vi "Validate XYZ limits.vi"(0 "X":sgl format="%.3g", 5 "Y":sgl format="%.3g", 7 "Z":sgl format="%.3g", 9 "Action":enum16{"Set Limit", "Validate limit"}(ring)=enum."Validate limit", 11 "error in (no error)":errorcluster, 12 "Controller ID":T1) -> (4 "Limit ok":bool, 15 "error out":errorcluster)   [LabVIEW 2024, in "GRBL 1.1.lvlib"]
doc: "This VI validate if new position requested is outside the limits."
uses:
  GRBL 1.1.lvlib
  Controller ID.ctl
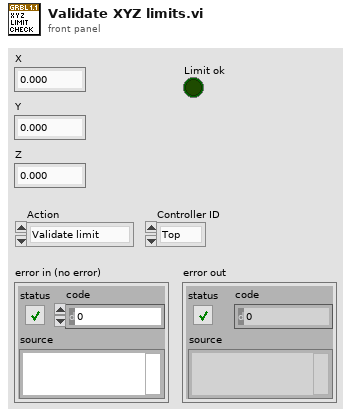
[diagram p1: front panel]
types:
  T1 = typedef "GRBL 1.1.lvlib/Controller ID.ctl" = enum16{"Top", "Bottom"}
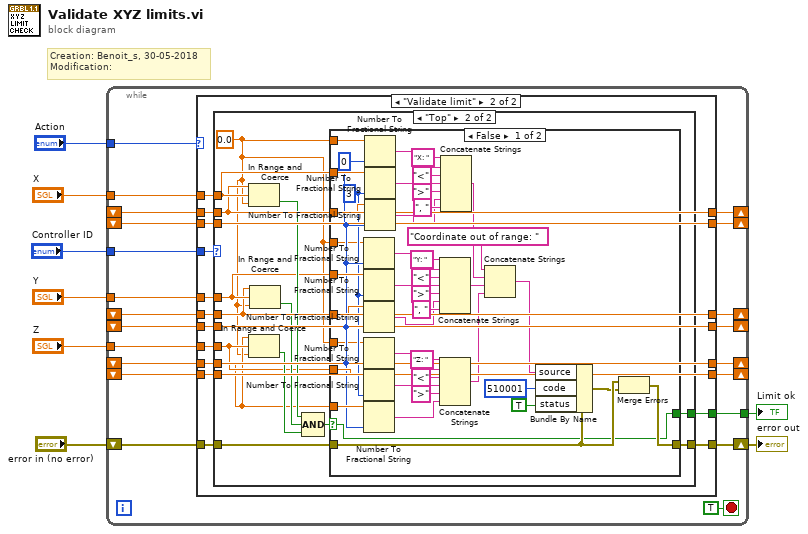
[diagram p0: block diagram]
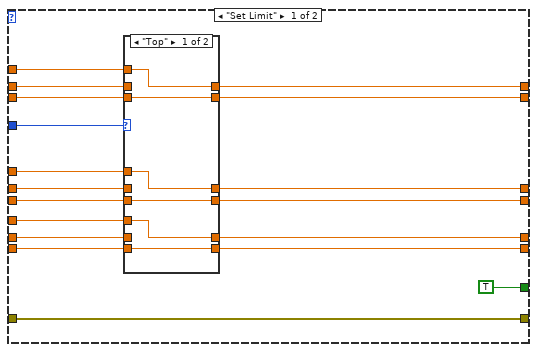
[diagram p2: hidden frame]
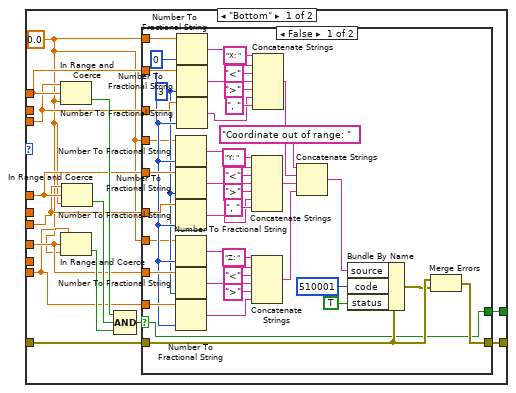
[diagram p4: hidden frame]
diagram:
  # "Creation: Benoit_s, 30-05-2018\nModification:"
  n1 = while {
    tunnel: "X" -> [w27]
    tunnel: "Y" -> [w26]
    tunnel: "Z" -> [w25]
    shift-right: [w28] -> w7
    shift-left: "error in (no error)" -> [w29]
    tunnel: [w23] -> w3
    tunnel: "Action" -> [w22]
    shift-right: [w18] -> _
    shift-left: _ -> [w21]
    shift-right: [w17] -> _
    shift-left: _ -> [w19]
    shift-right: [w16] -> _
    shift-left: _ -> [w20]
    tunnel: "Controller ID" -> [w15]
    shift-right: [w9] -> _
    shift-left: _ -> [w14]
    shift-right: [w10] -> _
    shift-left: _ -> [w13]
    shift-right: [w11] -> _
    shift-left: _ -> [w12]
    stop <- TRUE stop-if-true
    n2 = case shown="\"Validate limit\"" w22 {
      tunnel: w29 -> [w46 w72]
      tunnel: [w46 w71] -> w28
      tunnel: w27 -> [w43 w70]
      tunnel: w26 -> [w35 w69]
      tunnel: w25 -> [w33 w68]
      tunnel: [TRUE w67] -> w23
      tunnel: w21 -> [w32 w66]
      tunnel: w20 -> [w30 w64]
      tunnel: w19 -> [w31 w65]
      tunnel: [w44 w66] -> w18
      tunnel: [w36 w65] -> w17
      tunnel: [w34 w64] -> w16
      tunnel: w15 -> [w45 w63]
      tunnel: w14 -> [w37 w62]
      tunnel: w13 -> [w40 w61]
      tunnel: w12 -> [w41 w60]
      tunnel: [w42 w60] -> w11
      tunnel: [w39 w61] -> w10
      tunnel: [w38 w62] -> w9
      frame "Set Limit" {
        n3 = case shown="\"Top\"" w45 {
          tunnel: [w53 w58] -> w44
          tunnel: w43 -> [w53 w59]
          tunnel: [w52 w59] -> w42
          tunnel: w41 -> [w52 _]
          tunnel: w40 -> [w51 _]
          tunnel: [w51 w55] -> w39
          tunnel: [w50 w54] -> w38
          tunnel: w37 -> [w50 _]
          tunnel: [w49 w57] -> w36
          tunnel: w35 -> [w49 w55]
          tunnel: [w48 w56] -> w34
          tunnel: w33 -> [w48 w54]
          tunnel: w32 -> [_ w58]
          tunnel: w31 -> [_ w57]
          tunnel: w30 -> [_ w56]
          frame "Top" {
          }
          frame "Bottom" {
          }
        }
      }
      frame "Validate limit" {
        n4 = case shown="\"Top\"" w63 {
          tunnel: w72 -> [w82 w140]
          tunnel: [w81 w139] -> w71
          tunnel: w70 -> [w80 w138]
          tunnel: w69 -> [w79 w137]
          tunnel: w68 -> [w78 w136]
          tunnel: [w77 w135] -> w67
          tunnel: w66 -> [_ w134]
          tunnel: w65 -> [_ w133]
          tunnel: w64 -> [_ w132]
          tunnel: w60 -> [w76 _]
          tunnel: w62 -> [w74 _]
          tunnel: w61 -> [w75 _]
          frame "Bottom" {
            w73 = sgl 0.0 ("upper limit")
            n5 = In Range and Coerce(upper limit=w76, x=w80, lower limit=w73) -> (In Range?=w86:bool)  [unwired: 1 out]
            n6 = In Range and Coerce(upper limit=w74, x=w78, lower limit=w73) -> (In Range?=w84:bool)  [unwired: 1 out]
            n7 = In Range and Coerce(upper limit=w75, x=w79, lower limit=w73) -> (In Range?=w85:bool)  [unwired: 1 out]
            n8 = Compound Arithmetic op=AND(w86, w85, w84) -> (w83:bool)
            n9 = case shown="False" w83 {
              selector: w83 -> [w97 w129]
              tunnel: w82 -> [w100 w130]
              tunnel: [w98 w130] -> w81
              tunnel: w73 -> [w123 _]
              tunnel: w80 -> [w122 _]
              tunnel: w76 -> [w121 _]
              tunnel: w75 -> [w115 _]
              tunnel: w79 -> [w114 _]
              tunnel: w74 -> [w109 _]
              tunnel: w78 -> [w108 _]
              tunnel: [w97 w129] -> w77
              tunnel: w73 -> [w94 _]
              tunnel: w73 -> [w93 _]
              frame False {
                w95 = i16 3 ("precision (6)")
                w96 = i16 0 ("precision (6)")
                n10 = Number To Fractional String(number=w94, precision (6)=w96) -> (F-format string=w90:string)  [unwired: 2 in]
                n11 = Number To Fractional String(number=w114, precision (6)=w95) -> (F-format string=w116:string)  [unwired: 2 in]
                n12 = Number To Fractional String(number=w115, precision (6)=w96) -> (F-format string=w89:string)  [unwired: 2 in]
                n13 = Number To Fractional String(number=w93, precision (6)=w96) -> (F-format string=w88:string)  [unwired: 2 in]
                n14 = Number To Fractional String(number=w108, precision (6)=w95) -> (F-format string=w113:string)  [unwired: 2 in]
                n15 = Number To Fractional String(number=w109, precision (6)=w96) -> (F-format string=w87:string)  [unwired: 2 in]
                n16 = Number To Fractional String(number=w123, precision (6)=w96) -> (F-format string=w92:string)  [unwired: 2 in]
                n17 = Number To Fractional String(number=w122, precision (6)=w95) -> (F-format string=w128:string)  [unwired: 2 in]
                n18 = Number To Fractional String(number=w121, precision (6)=w96) -> (F-format string=w91:string)  [unwired: 2 in]
                n19 = Concatenate Strings("Y: " ("string"), w90, "<" ("string"), w116, ">" ("string"), w89, ", " ("string")) -> (w107:string)
                n20 = Concatenate Strings("Z: " ("string"), w88, "<" ("string"), w113, ">" ("string"), w87) -> (w105:string)
                n21 = Concatenate Strings("X: " ("string"), w92, "<" ("string"), w128, ">" ("string"), w91, ", " ("string")) -> (w106:string)
                n22 = Concatenate Strings("Coordinate out of range: ", w106, w107, w105) -> (w103:string)
                n23 = Bundle By Name(cluster=w100, "source"=w103, "code"=510001, "status"=TRUE) -> (w99:errorcluster)
                n24 = Merge Errors(w100, w99) -> (w98:errorcluster)
              }
              frame True {
              }
            }
          }
          frame "Top" {
            w131 = sgl 0.0 ("upper limit")
            n25 = In Range and Coerce(upper limit=w134, x=w138, lower limit=w131) -> (In Range?=w144:bool)  [unwired: 1 out]
            n26 = In Range and Coerce(upper limit=w132, x=w136, lower limit=w131) -> (In Range?=w142:bool)  [unwired: 1 out]
            n27 = In Range and Coerce(upper limit=w133, x=w137, lower limit=w131) -> (In Range?=w143:bool)  [unwired: 1 out]
            n28 = Compound Arithmetic op=AND(w144, w143, w142) -> (w141:bool)
            n29 = case shown="False" w141 {
              selector: w141 -> [w155 w187]
              tunnel: w140 -> [w158 w188]
              tunnel: [w156 w188] -> w139
              tunnel: w131 -> [w181 _]
              tunnel: w138 -> [w180 _]
              tunnel: w134 -> [w179 _]
              tunnel: w133 -> [w173 _]
              tunnel: w137 -> [w172 _]
              tunnel: w132 -> [w167 _]
              tunnel: w136 -> [w166 _]
              tunnel: [w155 w187] -> w135
              tunnel: w131 -> [w146 _]
              tunnel: w131 -> [w145 _]
              frame False {
                w153 = i16 3 ("precision (6)")
                w154 = i16 0 ("precision (6)")
                n30 = Number To Fractional String(number=w145, precision (6)=w154) -> (F-format string=w150:string)  [unwired: 2 in]
                n31 = Number To Fractional String(number=w172, precision (6)=w153) -> (F-format string=w174:string)  [unwired: 2 in]
                n32 = Number To Fractional String(number=w173, precision (6)=w154) -> (F-format string=w149:string)  [unwired: 2 in]
                n33 = Number To Fractional String(number=w146, precision (6)=w154) -> (F-format string=w148:string)  [unwired: 2 in]
                n34 = Number To Fractional String(number=w166, precision (6)=w153) -> (F-format string=w171:string)  [unwired: 2 in]
                n35 = Number To Fractional String(number=w167, precision (6)=w154) -> (F-format string=w147:string)  [unwired: 2 in]
                n36 = Number To Fractional String(number=w181, precision (6)=w154) -> (F-format string=w152:string)  [unwired: 2 in]
                n37 = Number To Fractional String(number=w180, precision (6)=w153) -> (F-format string=w186:string)  [unwired: 2 in]
                n38 = Number To Fractional String(number=w179, precision (6)=w154) -> (F-format string=w151:string)  [unwired: 2 in]
                n39 = Concatenate Strings("Y: " ("string"), w150, "<" ("string"), w174, ">" ("string"), w149, ", " ("string")) -> (w165:string)
                n40 = Concatenate Strings("Z: " ("string"), w148, "<" ("string"), w171, ">" ("string"), w147) -> (w163:string)
                n41 = Concatenate Strings("X: " ("string"), w152, "<" ("string"), w186, ">" ("string"), w151, ", " ("string")) -> (w164:string)
                n42 = Concatenate Strings("Coordinate out of range: ", w164, w165, w163) -> (w161:string)
                n43 = Bundle By Name(cluster=w158, "source"=w161, "code"=510001, "status"=TRUE) -> (w157:errorcluster)
                n44 = Merge Errors(w158, w157) -> (w156:errorcluster)
              }
              frame True {
              }
            }
          }
        }
      }
    }
  }
  "error out" <- w7
  "Limit ok" <- w3
